vi "WebSockets_Client.vi"() -> ()   [LabVIEW 2021]
uses:
  <vilib>/JDP Science/JSONtext/Next JSON Value.vi
  <vilib>/JDP Science/JSONtext/String Subset.vi
  <vilib>/JDP Science/JSONtext/Parsing/Advance past next JSON Value (inlined COPY).vi
  <vilib>/JDP Science/JSONtext/Parsing/Advance past whitespace.vi
  <vilib>/JDP Science/JSONtext/Parsing/Advance past String.vi
  <vilib>/JDP Science/JSONtext/Parsing/Advance past Number.vi
  <vilib>/JDP Science/JSONtext/Parsing/Advance past Line Ending.vi
  <vilib>/JDP Science/JSONtext/Parsing/Parse Full Path or Item Name.vi
  <vilib>/JDP Science/JSONtext/Parsing/Advance past Array.vi
  <vilib>/JDP Science/JSONtext/Parsing/Advance past Object.vi
  <vilib>/JDP Science/JSONtext/support/Error Cluster From Code.vi
  <vilib>/JDP Science/JSONtext/Offset/Find Item Locations by Path.vi
  <vilib>/MediaMongrels Ltd/WebSockets/WebSockets/WebSocket Client/WebSocket Client.lvclass
  <vilib>/JDP Science/JSONtext/JSONtext.lvlib
panel:
  out "ECG Chart":dbl(graph)
  in  "stop":bool
  in  "WebSocket URL":string="ws://192.168.10.115:81"
  in  "error in (no error)":errorcluster
  out "error out":errorcluster
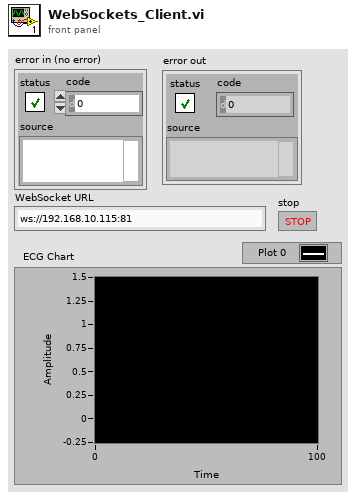
[diagram p1: front panel]
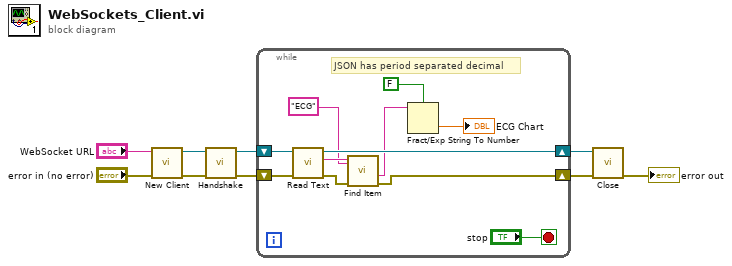
[diagram p0: block diagram]
diagram:
  n1 = call <vilib>:"New Client.vi"("error in (no error)"="error in (no error)", "WebSocket URL"="WebSocket URL") -> ("error out"=w9:errorcluster, "WebSocket Client out"=w8:refnum<class "WebSocket Client.lvclass">)  [unwired: 8 in]
  n2 = call-dynamic "Handshake.vi"("error in (no error)"=w9, "WebSocket Client in"=w8) -> ("error out"=w7:errorcluster, "WebSocket Client out"=w6:refnum<class "WebSocket Client.lvclass">)  [unwired: 8 in]
  n3 = while {
    shift-right: [w14] -> w1
    shift-left: w7 -> [w20]
    shift-right: [w18] -> w5
    shift-left: w6 -> [w19]
    stop <- "stop" stop-if-true
    # "JSON has period separated decimal"
    n4 = call-dynamic "Read Text.vi"("error in (no error)"=w20, "WebSocket in"=w19) -> ("error out"=w15:errorcluster, "Data"=w17:string, "WebSocket out"=w18:refnum<class "WebSocket Client.lvclass">)  [unwired: 7 in]
    n5 = call <vilib>:"Find Item.vi"("$Path or Item Name"="ECG", "error in (no error)"=w15, "JSON"=w17) -> ("error out"=w14:errorcluster, "<JSON>"=w13:string)  [unwired: 5 in, 2 out]
    n6 = Fract/Exp String To Number(use system decimal point (T)=FALSE, string=w13) -> (number=→"ECG Chart":dbl)  [unwired: 2 in, 1 out]
  }
  n7 = call-dynamic "Close.vi"("error in (no error)"=w1, "WebSocket in"=w5) -> ("error out"=→"error out":errorcluster)  [unwired: 9 in]
